vi "Create.vi"(10 "Groups":string[](array[string])) -> (3 "GroupsValue out":refnum<class "GroupNamesValue.lvclass">)   [LabVIEW 2020, in "Vecto.lvlib" / "GroupNamesValue.lvclass"]
uses:
  GroupNamesValue.lvclass
  GroupNamesValue.lvclass/GroupNamesValue.ctl
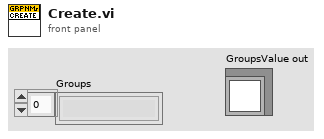
[diagram p1: front panel]
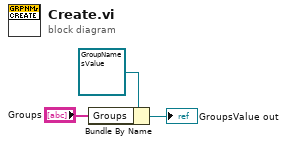
[diagram p0: block diagram]
diagram:
  n1 = Bundle By Name(cluster=refnum<class "GroupNamesValue.lvclass"> refnum ("GroupsValue out"), "Groups"="Groups") -> (→"GroupsValue out":refnum<class "GroupNamesValue.lvclass">)
